vi "Unpack Data.vi"(8 "error in (no error)":errorcluster, 10 "packed data size (bits)":i32, 11 "packed data in":i16[](array[numeric])) -> (0 "error out":errorcluster, 3 "unpacked data out":i16[](array[numeric]))   [LabVIEW 2021, in "Digitizer Control.lvclass"]
doc: "Unpacks an array of 16-bit integers containing a bit packed array of integers.\n\nInputs:\n\n<B>packed data in</B>: Array of I16s containing the packed data. The elements of the array are read LSB first.\n\n<B>packed data size (bits)</B>: The number of bits each <B>unpacked data out</B> array element should be written with.\n\nOutputs:\n\n<B>unpacked data out</B>: Array of integers containing the unpacked data. The elements of the array are written LSB first, then sign extended to 16 bits."
uses:
  Digitizer Control.lvclass
  <vilib>/Utility/error.llb/Error Cluster From Error Code.vi
  <vilib>/ErrorRing/Error Ring.xnode
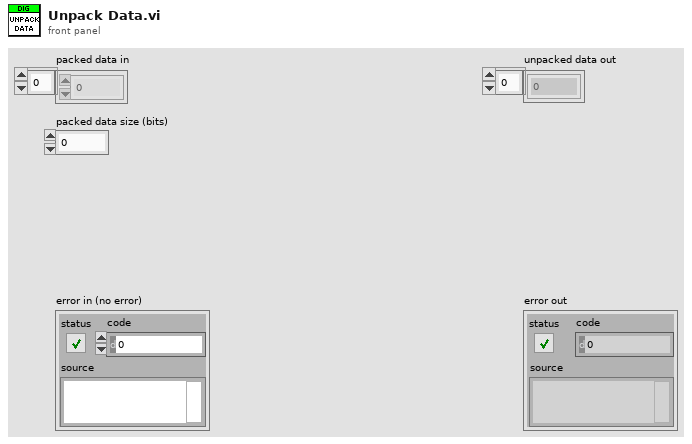
[diagram p1: front panel]
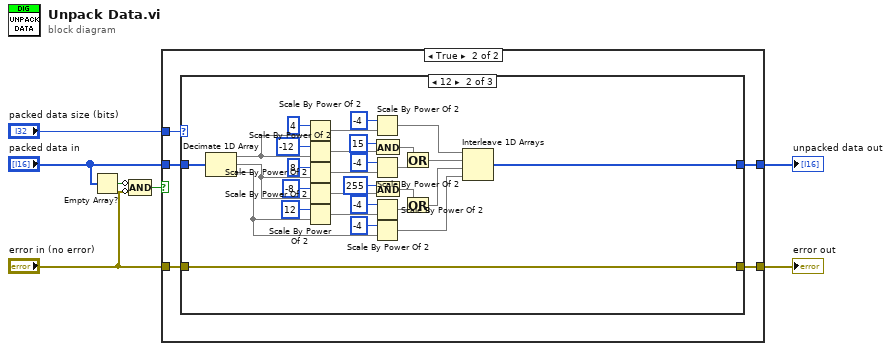
[diagram p0: block diagram]
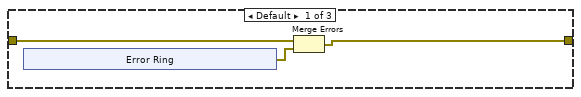
[diagram p3: hidden frame]
diagram:
  n1 = Empty Array?(array="packed data in") -> (empty?=w4:bool)
  n2 = Compound Arithmetic op=AND(invert w4, invert "error in (no error)") -> (w2:bool)
  n3 = case shown="True" w2 {
    tunnel: "packed data in" -> [_ w13]
    tunnel: "packed data size (bits)" -> [_ w12]
    tunnel: [_ w11] -> w6
    tunnel: [w8 w9] -> w5
    tunnel: "error in (no error)" -> [w8 w10]
    frame False {
    }
    frame True {
      n4 = case shown="12" w12 {
        tunnel: w10 -> [w16 w51 w53]
        tunnel: w13 -> [_ w50 w52]
        tunnel: [w14 w51 w53] -> w9
        tunnel: [_ w23 w52] -> w11
        frame Default {
          n5 = xnode "Error Ring"() -> ("error out"=w15:errorcluster)
          n6 = Merge Errors(w16, w15) -> (w14:errorcluster)
        }
        frame 12 {
          n7 = Decimate 1D Array(w50) -> (w47:i16[], w31:i16[], w28:i16[])
          n8 = Scale By Power Of 2(n=4, x=w47) -> (x*2^n=w22:i16[])
          n9 = Scale By Power Of 2(n=i16 -12 ("y"), x=w47) -> (x*2^n=w45:i16[])
          n10 = Scale By Power Of 2(n=8, x=w31) -> (x*2^n=w41:i16[])
          n11 = Scale By Power Of 2(n=i16 -8 ("y"), x=w31) -> (x*2^n=w33:i16[])
          n12 = Scale By Power Of 2(n=12, x=w28) -> (x*2^n=w36:i16[])
          n13 = Scale By Power Of 2(n=i16 -4 ("y"), x=w22) -> (x*2^n=w27:i16[])
          n14 = Scale By Power Of 2(n=i16 -4 ("y"), x=w41) -> (x*2^n=w39:i16[])
          n15 = Scale By Power Of 2(n=i16 -4 ("y"), x=w36) -> (x*2^n=w38:i16[])
          n16 = Scale By Power Of 2(n=i16 -4 ("y"), x=w28) -> (x*2^n=w24:i16[])
          n17 = And(x=i16 15, y=w45) -> (x .and. y?=w40:i16[])
          n18 = And(x=i16 255, y=w33) -> (x .and. y?=w37:i16[])
          n19 = Or(x=w40, y=w39) -> (x .or. y?=w26:i16[])
          n20 = Or(x=w37, y=w38) -> (x .or. y?=w25:i16[])
          n21 = Interleave 1D Arrays(w27, w26, w25, w24) -> (w23:i16[])
        }
        frame 16 {
        }
      }
    }
  }
  "error out" <- w5
  "unpacked data out" <- w6
